vi "PI_22.vi"(7 "SLMAX":fxp<+/-,18,5>, 10 "ziyi_f_in":T1=[0.0, 0.0, 0.0, 0.0, 0.0, 0.0, 0.0, 0.0, 0.0, 0.0, 0.0, 0.0, 0.0, 0.0, 0.0, 0.0, 0.0, 0.0, 0.0, 0.0, 0.0, 0.0]) -> (2 "ziyi_f_out":T1)   [LabVIEW 2017]
uses:
  ziyi_pipe_N22.ctl
  x_qp_scalar.ctl
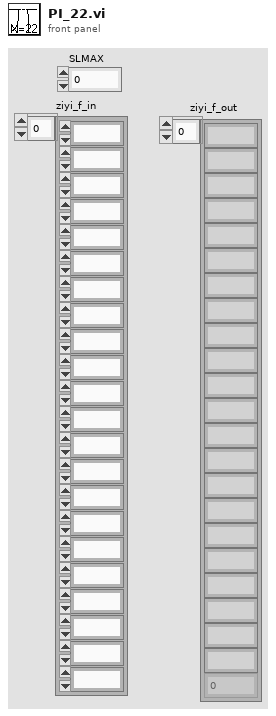
[diagram p1: front panel]
types:
  T1 = typedef "ziyi_pipe_N22.ctl" = T2[]
  T2 = typedef "x_qp_scalar.ctl" = fxp<+/-,32,6>
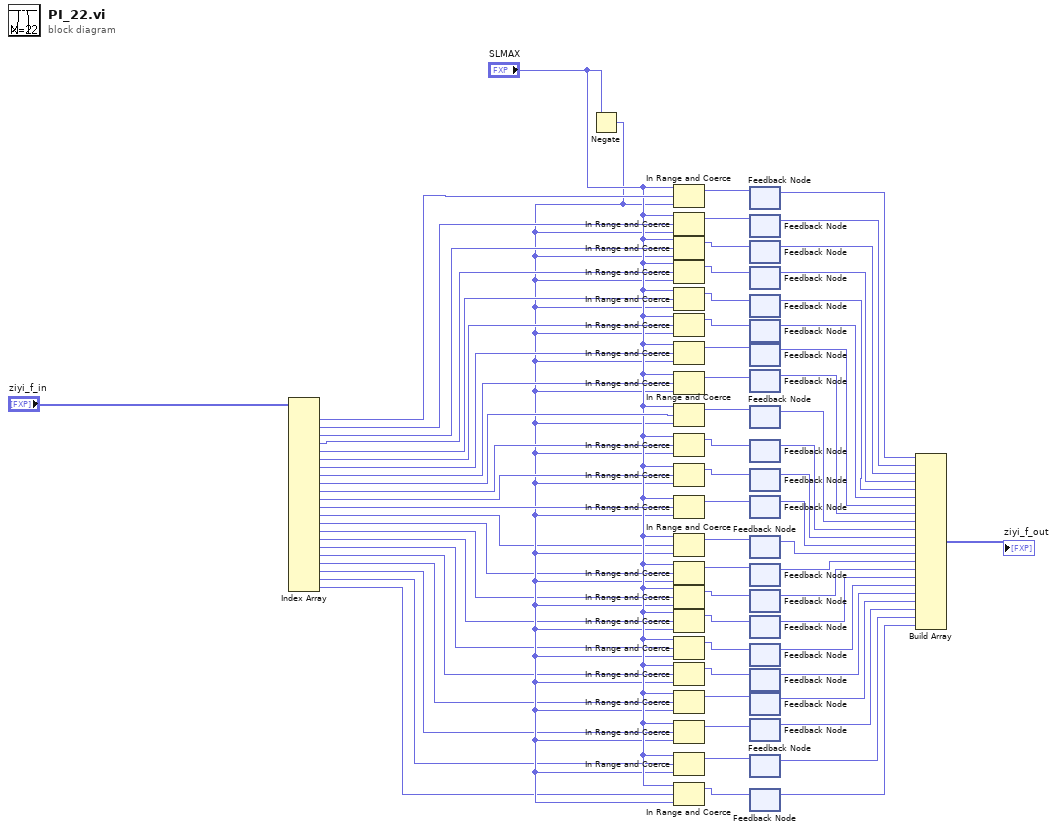
[diagram p0: block diagram]
diagram:
  n1 = Index Array(array="ziyi_f_in") -> (element #1=w46:T2, element #2=w45:T2, element #3=w44:T2, element #4=w43:T2, element #5=w42:T2, element #6=w41:T2, element #7=w40:T2, element #8=w39:T2, element #9=w38:T2, element #10=w37:T2, element #11=w36:T2, element #12=w35:T2, element #13=w20:T2, element #14=w19:T2, element #15=w18:T2, element #16=w17:T2, element #17=w16:T2, element #18=w15:T2, element #19=w14:T2, element #20=w13:T2, element #21=w12:T2, element #22=w11:T2)  [unwired: 22 in]
  n2 = Negate(x="SLMAX") -> (-x=w21:fxp<+/-,18,4>)
  n3 = In Range and Coerce(upper limit="SLMAX", x=w46, lower limit=w21) -> (coerced(x)=w70:T2)  [unwired: 1 out]
  n4 = In Range and Coerce(upper limit="SLMAX", x=w45, lower limit=w21) -> (coerced(x)=w69:T2)  [unwired: 1 out]
  n5 = In Range and Coerce(upper limit="SLMAX", x=w44, lower limit=w21) -> (coerced(x)=w68:T2)  [unwired: 1 out]
  n6 = In Range and Coerce(upper limit="SLMAX", x=w43, lower limit=w21) -> (coerced(x)=w67:T2)  [unwired: 1 out]
  n7 = In Range and Coerce(upper limit="SLMAX", x=w42, lower limit=w21) -> (coerced(x)=w66:T2)  [unwired: 1 out]
  n8 = In Range and Coerce(upper limit="SLMAX", x=w41, lower limit=w21) -> (coerced(x)=w65:T2)  [unwired: 1 out]
  n9 = In Range and Coerce(upper limit="SLMAX", x=w40, lower limit=w21) -> (coerced(x)=w64:T2)  [unwired: 1 out]
  n10 = In Range and Coerce(upper limit="SLMAX", x=w39, lower limit=w21) -> (coerced(x)=w63:T2)  [unwired: 1 out]
  n11 = In Range and Coerce(upper limit="SLMAX", x=w38, lower limit=w21) -> (coerced(x)=w62:T2)  [unwired: 1 out]
  n12 = In Range and Coerce(upper limit="SLMAX", x=w37, lower limit=w21) -> (coerced(x)=w61:T2)  [unwired: 1 out]
  n13 = In Range and Coerce(upper limit="SLMAX", x=w36, lower limit=w21) -> (coerced(x)=w60:T2)  [unwired: 1 out]
  n14 = In Range and Coerce(upper limit="SLMAX", x=w35, lower limit=w21) -> (coerced(x)=w59:T2)  [unwired: 1 out]
  n15 = In Range and Coerce(upper limit="SLMAX", x=w20, lower limit=w21) -> (coerced(x)=w32:T2)  [unwired: 1 out]
  n16 = In Range and Coerce(upper limit="SLMAX", x=w19, lower limit=w21) -> (coerced(x)=w31:T2)  [unwired: 1 out]
  n17 = In Range and Coerce(upper limit="SLMAX", x=w18, lower limit=w21) -> (coerced(x)=w30:T2)  [unwired: 1 out]
  n18 = In Range and Coerce(upper limit="SLMAX", x=w17, lower limit=w21) -> (coerced(x)=w29:T2)  [unwired: 1 out]
  n19 = In Range and Coerce(upper limit="SLMAX", x=w16, lower limit=w21) -> (coerced(x)=w28:T2)  [unwired: 1 out]
  n20 = In Range and Coerce(upper limit="SLMAX", x=w15, lower limit=w21) -> (coerced(x)=w27:T2)  [unwired: 1 out]
  n21 = In Range and Coerce(upper limit="SLMAX", x=w14, lower limit=w21) -> (coerced(x)=w26:T2)  [unwired: 1 out]
  n22 = In Range and Coerce(upper limit="SLMAX", x=w13, lower limit=w21) -> (coerced(x)=w25:T2)  [unwired: 1 out]
  n23 = In Range and Coerce(upper limit="SLMAX", x=w12, lower limit=w21) -> (coerced(x)=w24:T2)  [unwired: 1 out]
  n24 = In Range and Coerce(upper limit="SLMAX", x=w11, lower limit=w21) -> (coerced(x)=w23:T2)  [unwired: 1 out]
  n25 = feedback #1() -> (w58:T2)  [unwired: 1 in]
  n26 = feedback-in #1(w70) -> ()
  n27 = feedback #2() -> (w57:T2)  [unwired: 1 in]
  n28 = feedback-in #2(w69) -> ()
  n29 = feedback #3() -> (w56:T2)  [unwired: 1 in]
  n30 = feedback-in #3(w68) -> ()
  n31 = feedback #4() -> (w55:T2)  [unwired: 1 in]
  n32 = feedback-in #4(w67) -> ()
  n33 = feedback #5() -> (w54:T2)  [unwired: 1 in]
  n34 = feedback-in #5(w66) -> ()
  n35 = feedback #6() -> (w53:T2)  [unwired: 1 in]
  n36 = feedback-in #6(w65) -> ()
  n37 = feedback #7() -> (w52:T2)  [unwired: 1 in]
  n38 = feedback-in #7(w64) -> ()
  n39 = feedback #8() -> (w51:T2)  [unwired: 1 in]
  n40 = feedback-in #8(w63) -> ()
  n41 = feedback #9() -> (w50:T2)  [unwired: 1 in]
  n42 = feedback-in #9(w62) -> ()
  n43 = feedback #10() -> (w49:T2)  [unwired: 1 in]
  n44 = feedback-in #10(w61) -> ()
  n45 = feedback #11() -> (w48:T2)  [unwired: 1 in]
  n46 = feedback-in #11(w60) -> ()
  n47 = feedback #12() -> (w47:T2)  [unwired: 1 in]
  n48 = feedback-in #12(w59) -> ()
  n49 = feedback #13() -> (w10:T2)  [unwired: 1 in]
  n50 = feedback-in #13(w32) -> ()
  n51 = feedback #14() -> (w9:T2)  [unwired: 1 in]
  n52 = feedback-in #14(w31) -> ()
  n53 = feedback #15() -> (w8:T2)  [unwired: 1 in]
  n54 = feedback-in #15(w30) -> ()
  n55 = feedback #16() -> (w7:T2)  [unwired: 1 in]
  n56 = feedback-in #16(w29) -> ()
  n57 = feedback #17() -> (w6:T2)  [unwired: 1 in]
  n58 = feedback-in #17(w28) -> ()
  n59 = feedback #18() -> (w5:T2)  [unwired: 1 in]
  n60 = feedback-in #18(w27) -> ()
  n61 = feedback #19() -> (w4:T2)  [unwired: 1 in]
  n62 = feedback-in #19(w26) -> ()
  n63 = feedback #20() -> (w3:T2)  [unwired: 1 in]
  n64 = feedback-in #20(w25) -> ()
  n65 = feedback #21() -> (w2:T2)  [unwired: 1 in]
  n66 = feedback-in #21(w24) -> ()
  n67 = feedback #22() -> (w1:T2)  [unwired: 1 in]
  n68 = feedback-in #22(w23) -> ()
  n69 = Build Array(w58, w57, w56, w55, w54, w53, w52, w51, w50, w49, w48, w47, w10, w9, w8, w7, w6, w5, w4, w3, w2, w1) -> (→"ziyi_f_out":T2[])
